vi "StopCore.vi"(8 "error in (no error)":errorcluster, 11 "MicronClient in":refnum<class "MicronClient.lvclass">) -> (0 "error out":errorcluster, 2 "Response":string, 3 "MicronClient out":refnum<class "MicronClient.lvclass">)   [LabVIEW 2019, in "MicronClient.lvclass"]
uses:
  MicronClient.lvclass
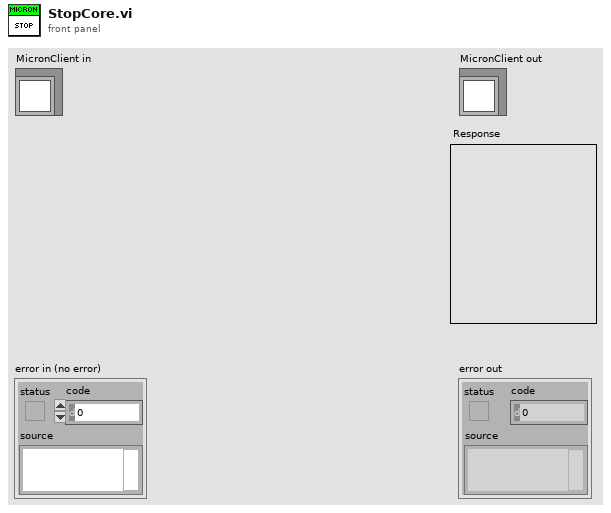
[diagram p1: front panel]
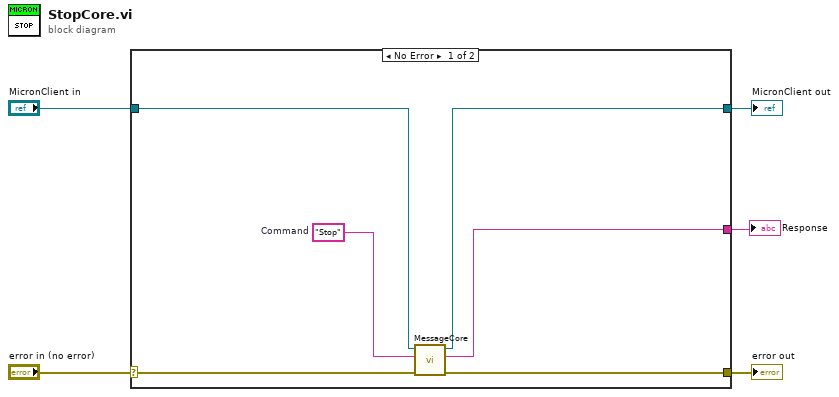
[diagram p0: block diagram]
diagram:
  n1 = case shown="No Error" "error in (no error)" {
    selector: "error in (no error)" -> [w11 w13]
    tunnel: [w10 w13] -> w4
    tunnel: [w8 w12] -> w2
    tunnel: "MicronClient in" -> [w9 w12]
    tunnel: [w6 _] -> w1
    frame No Error {
      w7 = "Stop"  # Command
      n2 = call-dynamic "MessageCore.vi"("error in (no error)"=w11, "Command"=w7, "MicronClient in"=w9) -> ("error out"=w10:errorcluster, "Response"=w6:string, "MicronClient out"=w8:refnum<class "MicronClient.lvclass">)  [unwired: 6 in]
    }
    frame Error {
    }
  }
  "error out" <- w4
  "MicronClient out" <- w2
  "Response" <- w1
